vi "populateArrays_sub_analog.vi"(11 "Instance":i32) -> (2 "ADC_Array":dbl[](array[numeric]))   [LabVIEW 2022 SP3]
uses:
  LVLib/SADI_FW3.lvlib
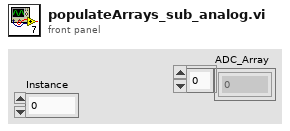
[diagram p1: front panel]
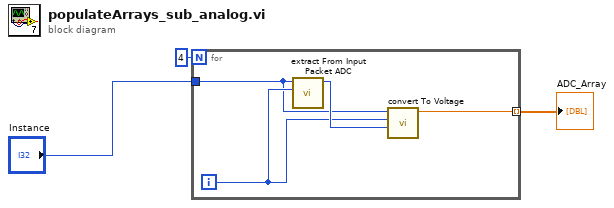
[diagram p0: block diagram]
diagram:
  n1 = for {
    N: 4 -> [_]
    tunnel: [w5] -> w2 mode=indexing
    tunnel: "Instance" -> [w4]
    i -> [w6]
    n2 = call "extract From Input Packet ADC.vi"("channel"=w6, "instance"=w4) -> ("function return"=w7:i16)  [unwired: 9 in]
    n3 = call "convert To Voltage.vi"("value"=w7, "adcCh"=w6, "instance"=w4) -> ("function return"=w5:dbl)  [unwired: 8 in]
  }
  "ADC_Array" <- w2
